vi "getParallelSpeed.vi"(6 "Delay between send and receive [ms]":i32=100, 8 "error in (no error)":errorcluster, 11 "CCD in":refnum<class "CCD.lvclass">) -> (0 "error out":errorcluster, 1 "token":i32, 2 "info":string, 3 "CCD out":refnum<class "CCD.lvclass">)   [LabVIEW 2023, in "horiba.lvlib" / "CCD.lvclass"]
doc: "Gets the current parallel speed token and token description. Parallel speed tokens and their descriptions are contained in the CCD configuration information. See ccd_getConfig command.\n\nNote: The Parallel Speed value may also be referred to as the Vertical Shift Rate. These terms are interchangeable.\n\nFor example:\n\n\"parallelSpeeds\": [\n {\n \"info\": \"9.6 µSec\",\n \"token\": 1\n },\n {\n \"info\": \"4.9 µSec\",\n \"token\": 2\n },\n {\n \"info\": \"19 µSec\",\n \"token\": 0\n }\n],"
uses:
  CCD.lvclass
  Speed.ctl
  20f7d3bd-08ac-4524-9bed-df36c1da25a0.vi
  a21955fc-e3a0-4e36-8495-41f1bfac7860.vi
  <vilib>/JDP Science/JSONtext/Variant to JSON Text.vi
  <vilib>/JDP Science/JSONtext/Set Item.vi
  <vilib>/JDP Science/JSONtext/JSON text to Variant.vi
  <vilib>/JDP Science/JSONtext/LVClass Serializer/JSONtext LVClass Serializer.lvclass
  CCD.lvclass/CCD.ctl
  GenericDevice/GenericDevice.lvclass
  <vilib>/JDP Science/JSONtext/JSONtext.lvlib
panel:
  # "Connector Pane"
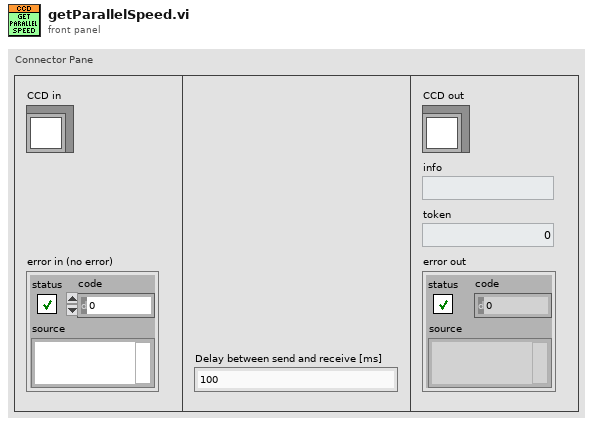
[diagram p1: front panel]
types:
  T1 = typedef "horiba.lvlib/CCD.lvclass/Speed.ctl" = cluster{"info":string, "token":i32}
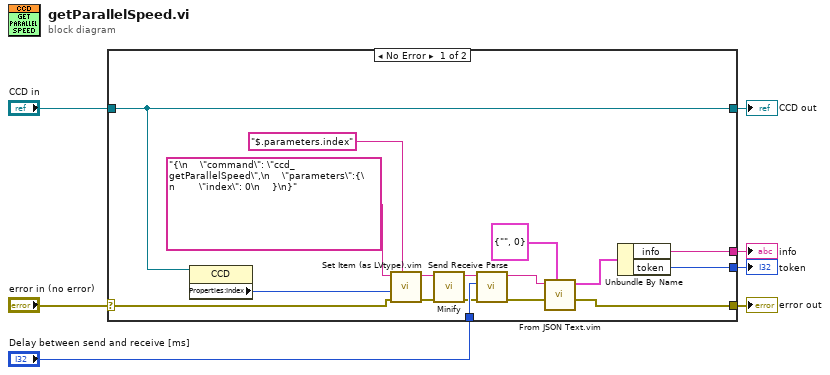
[diagram p0: block diagram]
diagram:
  n1 = case shown="No Error" "error in (no error)" {
    selector: "error in (no error)" -> [w20 w26]
    tunnel: [w19 w26] -> w6
    tunnel: [w22 w25] -> w4
    tunnel: "CCD in" -> [w22 w25]
    tunnel: [w14 _] -> w3
    tunnel: [w12 _] -> w1
    tunnel: "Delay between send and receive [ms]" -> [w13 _]
    frame No Error {
      n2 = property class="CCD"(reference=w22) -> ("Properties:Index"=w21:i32)  [unwired: 1 in, 2 out]
      n3 = call "Set Item (as LVtype).vim"("$Path or Item Name"="$.parameters.index", "error in (no error)"=w20, "Anything"=w21, "JSON"="{\n    \"command\": \"ccd_getParallelSpeed\",\n    \"parameters\":{\n        \"index\": 0\n    }\n}") -> ("error out"=w17:errorcluster, "<JSON>"=w9:string)  [unwired: 4 in, 1 out]
      n4 = call <vilib>:"Minify.vi"("error in (no error)"=w17, "JSON"=w9) -> ("error out"=w10:errorcluster, "<JSON>"=w8:string)  [unwired: 7 in, 1 out]
      n5 = call "Send Receive Parse.vi"("error in"=w10, "Delay between send and receive [ms]"=w13, "<JSON>"=w8) -> ("error out"=w16:errorcluster, "results-JSON string"=w18:string)  [unwired: 6 in, 1 out]
      n6 = call "From JSON Text.vim"("Data Type and Default Value"=T1 {"info"="", "token"=0} ("speed"), "error in (no error)"=w16, "JSON"=w18) -> ("error out"=w19:errorcluster, "Data out"=w15:T1)  [unwired: 7 in]
      n7 = Unbundle By Name(w15) -> ("info"=w14:string, "token"=w12:i32)
    }
    frame Error {
    }
  }
  "error out" <- w6
  "CCD out" <- w4
  "info" <- w3
  "token" <- w1
